vi "Filter.vi"(9 "FilterSpecification":refnum<class "IFilterSpecification.lvclass">, 10 "Products In":refnum<class "Product.lvclass">[](array[class]), 11 "IFilter":refnum<class "IFilter.lvclass">) -> (2 "Filtered Products":refnum<class "Product.lvclass">[](array[class]))   [LabVIEW 2018, in "IFilter.lvclass"]
uses:
  IFilter.lvclass
  IFilterSpecification/IFilterSpecification.lvclass
  Product/Product.lvclass
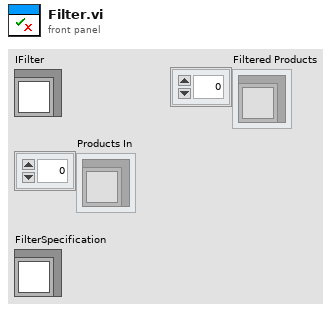
[diagram p1: front panel]
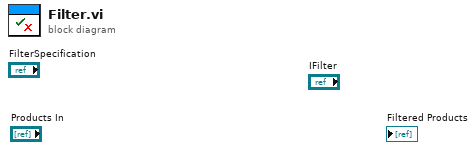
[diagram p0: block diagram]
diagram:
